vi "OA Get Number Of Acq Params.vi"(10 "puiNumberOfParams":u32, 11 "pcModeName":string) -> (2 "puiNumberOfParams out":u32, 3 "function return":u32)   [LabVIEW 2018, in "AndorSDK.lvlib"]
doc: "EXPNETTYPE unsigned int WINAPI OA_GetNumberOfAcqParams(const char * const pcModeName, unsigned int * const puiNumberOfParams);"
uses:
  AndorSDK.lvlib
  ATMCD32D.dll
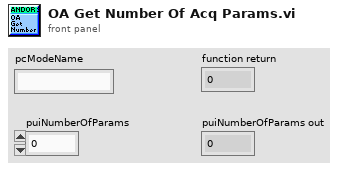
[diagram p1: front panel]
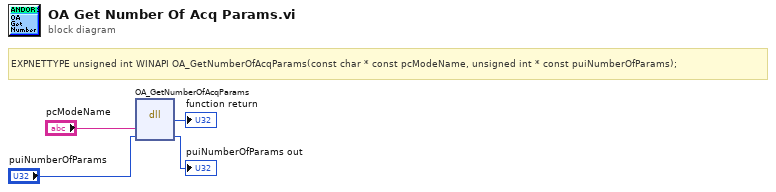
[diagram p0: block diagram]
diagram:
  # "EXPNETTYPE unsigned int WINAPI OA_GetNumberOfAcqParams(const char * const pcModeName, unsigned int * const puiNumberOfParams);"
  n1 = dll-call lib="PTH2babs E\nPersönliches02 - Arbeit03-HiwijobsLabviewCodelibANDOR\tAndor SDK\nATMCD32D.*" fn="OA_GetNumberOfAcqParams"("pcModeName"="pcModeName", "puiNumberOfParams"="puiNumberOfParams") -> (→"function return":u32, "puiNumberOfParams"=→"puiNumberOfParams out":u32)  [unwired: 4 in, 2 out]
